vi "ResetStreamingFilter.Do.vi"(8 "error in (no error)":errorcluster, 10 "State Variables":T2, 11 "gRPC Request":T1) -> (0 "error out":errorcluster, 2 "State Variables out":T2, 3 "gRPC Response":T13)   [LabVIEW 2025, in "xnet_can_bus_monitor_api_server_do.lvlib"]
uses:
  xnet_can_bus_monitor_api_server_do.lvlib
  xnet_can_bus_monitor_api_server/RPC Messages/ni_xnet_can_bm_api_ErrorInfo.ctl
  xnet_can_bus_monitor_api_server/xnet_can_bus_monitor_api_server.lvlib
  xnet_can_bus_monitor_api_server/RPC Messages/ni_xnet_can_bm_api_FrameFilter.ctl
  xnet_can_bus_monitor_api_server/RPC Messages/ni_xnet_can_bm_api_DirectionFilter.ctl
  xnet_can_bus_monitor_api_server/RPC Messages/ni_xnet_can_bm_api_FilterInfo.ctl
  xnet_can_bus_monitor_api_server/RPC Messages/ni_xnet_can_bm_api_ResetStreamingFilterReply.ctl
  xnet_can_bus_monitor_api_server/RPC Messages/ni_xnet_can_bm_api_FdIsoMode.ctl
  xnet_can_bus_monitor_api_server/RPC Messages/ni_xnet_can_bm_api_Termination.ctl
  xnet_can_bus_monitor_api_server/RPC Messages/ni_xnet_can_bm_api_CanMode.ctl
  xnet_can_bus_monitor_api_server/RPC Messages/ni_xnet_can_bm_api_ConnectSettings.ctl
  Types/XNET.InitialSettings.ctl
  Types/StreamProcess.VIRef.ctl
  Types/StreamProcess.Refs.ctl
  Types/MainProcess.StateVariables.ctl
  xnet_can_bus_monitor_api_server/RPC Messages/ni_xnet_can_bm_api_ResetStreamingFilterRequest.ctl
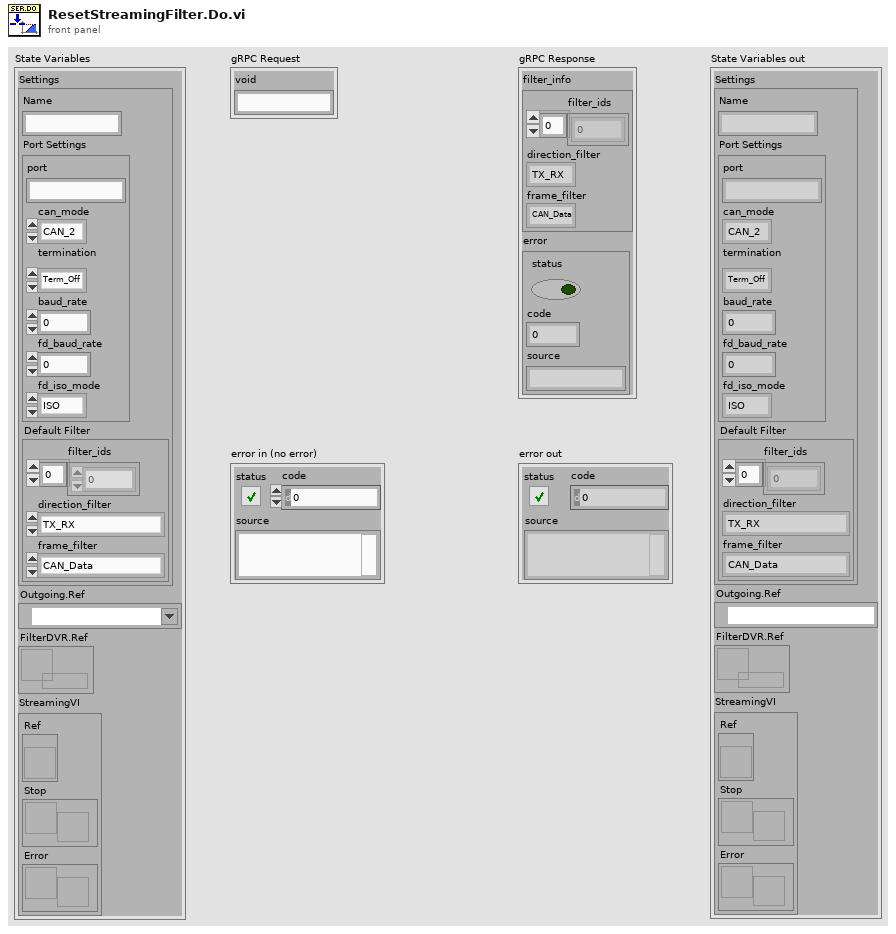
[diagram p1: front panel]
types:
  T1 = typedef "xnet_can_bus_monitor_api_server.lvlib/ni_xnet_can_bm_api_ResetStreamingFilterRequest.ctl" = cluster{"void":string}
  T2 = typedef "xnet_can_bus_monitor_api_server_do.lvlib/MainProcess.StateVariables.ctl" = cluster{"Settings":T3, "Outgoing.Ref":refnum<k21>, "FilterDVR.Ref":refnum<data-value>, "StreamingVI":T11}
  T3 = typedef "xnet_can_bus_monitor_api_server_do.lvlib/XNET.InitialSettings.ctl" = cluster{"Name":string, "Port Settings":T4, "Default Filter":T8}
  T4 = typedef "xnet_can_bus_monitor_api_server.lvlib/ni_xnet_can_bm_api_ConnectSettings.ctl" = cluster{"port":string, "can_mode":T5, "termination":T6, "baud_rate":u64, "fd_baud_rate":u64, "fd_iso_mode":T7}
  T5 = typedef "xnet_can_bus_monitor_api_server.lvlib/ni_xnet_can_bm_api_CanMode.ctl" = enum32{"CAN_2", "CAN_FD", "CAN_FD_BRS"}
  T6 = typedef "xnet_can_bus_monitor_api_server.lvlib/ni_xnet_can_bm_api_Termination.ctl" = enum32{"Term_Off", "Term_On"}
  T7 = typedef "xnet_can_bus_monitor_api_server.lvlib/ni_xnet_can_bm_api_FdIsoMode.ctl" = enum32{"ISO", "Non_ISO", "ISO_Legacy"}
  T8 = typedef "xnet_can_bus_monitor_api_server.lvlib/ni_xnet_can_bm_api_FilterInfo.ctl" = cluster{"filter_ids":u32[], "direction_filter":T9, "frame_filter":T10}
  T9 = typedef "xnet_can_bus_monitor_api_server.lvlib/ni_xnet_can_bm_api_DirectionFilter.ctl" = enum32{"TX_RX", "RX", "TX"}
  T10 = typedef "xnet_can_bus_monitor_api_server.lvlib/ni_xnet_can_bm_api_FrameFilter.ctl" = enum32{"CAN_Data", "CAN_Remote", "CAN_Bus_Error", "CAN_2_Data", "CAN_FD_Data", "CAN_FD_BRS_Data", "J1939_Data", "Delay", "Log_Trigger", "Start_Trigger", "All"}
  T11 = typedef "xnet_can_bus_monitor_api_server_do.lvlib/StreamProcess.Refs.ctl" = cluster{"Ref":T12, "Stop":refnum<notifier>, "Error":refnum<notifier>}
  T12 = typedef "xnet_can_bus_monitor_api_server_do.lvlib/StreamProcess.VIRef.ctl" = refnum<vi>
  T13 = typedef "xnet_can_bus_monitor_api_server.lvlib/ni_xnet_can_bm_api_ResetStreamingFilterReply.ctl" = cluster{"filter_info":T8, "error":T14}
  T14 = typedef "xnet_can_bus_monitor_api_server.lvlib/ni_xnet_can_bm_api_ErrorInfo.ctl" = errorcluster
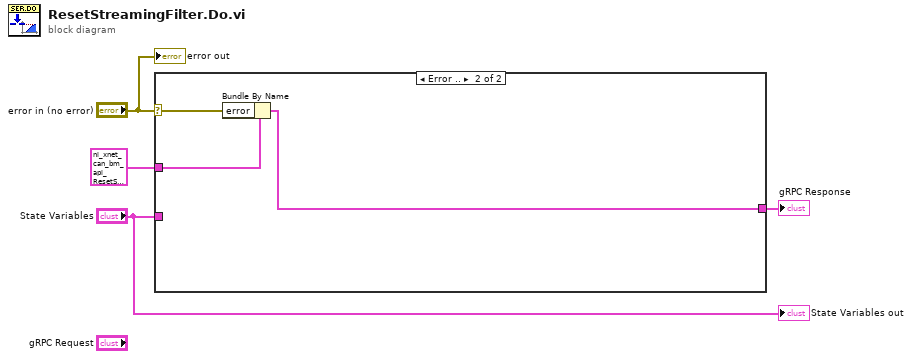
[diagram p0: block diagram]
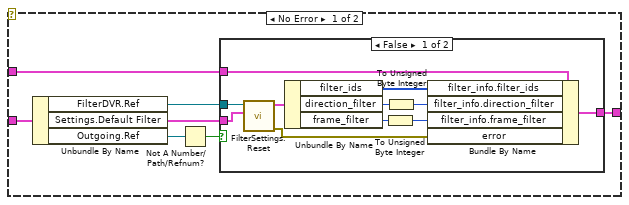
[diagram p2: hidden frame]
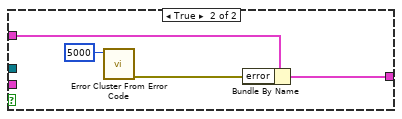
[diagram p3: hidden frame]
diagram:
  n1 = case shown="Error .." "error in (no error)" {
    selector: "error in (no error)" -> [_ w28]
    tunnel: "State Variables" -> [w8 _]
    tunnel: [w6 w27] -> w3
    tunnel: T13 {"filter_info"={"filter_ids"=[], "direction_filter"=enum."TX_RX", "frame_filter"=enum."CAN_Data"}, "error"={"status"=FALSE, "code"=0, "source"=""}} ("Message Data") -> [w5 w29]
    frame No Error {
      n2 = Unbundle By Name(w8) -> ("FilterDVR.Ref"=w11:refnum<data-value>, "Settings.Default Filter"=w10:T8, "Outgoing.Ref"=w9:refnum<k21>)
      n3 = Not A Number/Path/Refnum?(number/path/refnum=w9) -> (NaN/Path/Refnum?=w7:bool)
      n4 = case shown="False" w7 {
        tunnel: w11 -> [w22 _]
        tunnel: w5 -> [w21 w26]
        tunnel: [w15 w25] -> w6
        tunnel: w10 -> [w12 _]
        frame False {
          n5 = call "FilterSettings.Reset.vi"("Default Filter"=w12, "FilterDVR.Ref"=w22) -> ("error out"=w16:errorcluster, "Filter"=w20:T8)  [unwired: 8 in]
          n6 = Unbundle By Name(w20) -> ("filter_ids"=w19:u32[], "direction_filter"=w18:T9, "frame_filter"=w17:T10)
          n7 = To Unsigned Byte Integer(number=w17) -> (unsigned 8bit integer=w14:u8)
          n8 = To Unsigned Byte Integer(number=w18) -> (unsigned 8bit integer=w13:u8)
          n9 = Bundle By Name(cluster=w21, "filter_info.filter_ids"=w19, "filter_info.direction_filter"=w13, "filter_info.frame_filter"=w14, "error"=w16) -> (w15:T13)
        }
        frame True {
          n10 = call <vilib>:"Error Cluster From Error Code.vi"("error code (0)"=5000) -> ("error out"=w23:errorcluster)  [unwired: 8 in]
          n11 = Bundle By Name(cluster=w26, "error"=w23) -> (w25:T13)
        }
      }
    }
    frame Error {
      n12 = Bundle By Name(cluster=w29, "error"=w28) -> (w27:T13)
    }
  }
  "gRPC Response" <- w3
  "State Variables out" <- "State Variables"
  "error out" <- "error in (no error)"
